vi "Test_Create_ARGB.vi"(8 "error in (no error)":errorcluster, 11 "Test Case In":refnum<class "Image.lvclass">) -> (0 "error out":errorcluster, 3 "Test Case Out":refnum<class "Image.lvclass">)   [LabVIEW 2020, in "g_ar_toolkit.test.lvlib" / "Image.lvclass"]
uses:
  Image.lvclass
  Image.lvclass/Image.ctl
  g_ar_toolkit.image/g_ar_toolkit.image.lvlib
  g_ar_toolkit.image/CreateEmptyImageARGB.vi
  g_ar_toolkit.image/ARGB Colour.ctl
  g_ar_toolkit.image/Image Size (Fixed).ctl
  4993e8ee-a06a-463a-9684-69129f64d5ce.vi
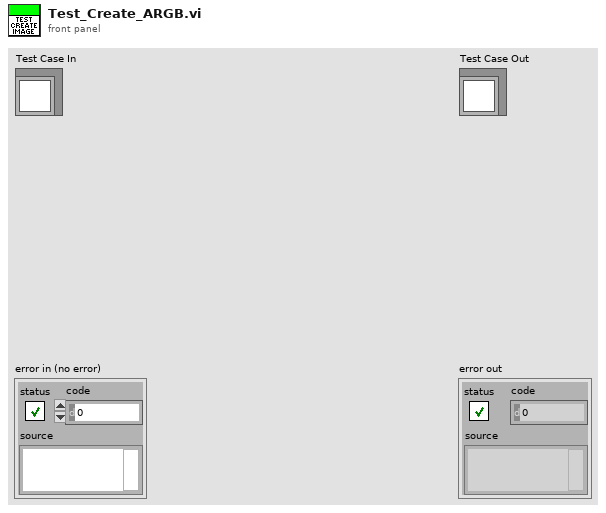
[diagram p1: front panel]
types:
  T1 = typedef "g_ar_toolkit.image.lvlib/Image Size (Fixed).ctl" = cluster{"Width":u16, "Height":u16}
  T2 = typedef "g_ar_toolkit.image.lvlib/ARGB Colour.ctl" = cluster{"Alpha":u8, "RGB":u32}
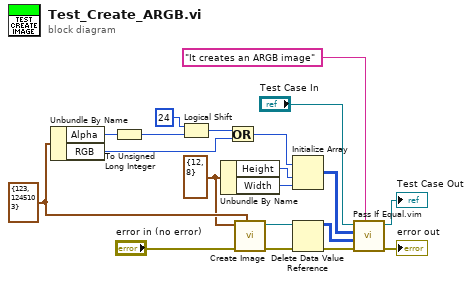
[diagram p0: block diagram]
diagram:
  w6 = T1 {"Width"=12, "Height"=8} ("Preallocated Image Size (Default: 0,0)")
  w13 = T2 {"Alpha"=123, "RGB"=1245103} ("Colour (Default: Black)")
  n1 = Unbundle By Name(w13) -> ("Alpha"=w11:u8, "RGB"=w12:u32)
  n2 = To Unsigned Long Integer(number=w11) -> (unsigned 32bit integer=w8:u32)
  n3 = Logical Shift(y=i16 24, x=w8) -> (x << y=w9:u32)
  n4 = Unbundle By Name(w6) -> ("Height"=w5:u16, "Width"=w4:u16)
  n5 = Or(x=w9, y=w12) -> (x .or. y?=w7:u32)
  n6 = call-poly "Create Image.vi"("Colour (Default: Black)"=w13, "error in (no error)"="error in (no error)", "Preallocated Image Size (Default: 0,0)"=w6) -> ("error out"=w15:errorcluster, "New ARGB Image"=w16:refnum<data-value>)  [unwired: 7 in]
  n7 = Initialize Array(w7, w5, w4) -> (w3:u32[][])
  n8 = Delete Data Value Reference(data value reference=w16, error in=w15) -> (data value=w2:u32[][], error out=w14:errorcluster)
  n9 = call "Pass If Equal.vim"("Description"="It creates an ARGB image", "error in (no error)"=w14, "Actual"=w2, "Expected"=w3, "LUnit Test Case In"="Test Case In") -> ("error out"=→"error out":errorcluster, "LUnit Test Case Out"=→"Test Case Out":refnum<class "Image.lvclass">)  [unwired: 5 in]
